vi "main_DMM.vi"() -> ()   [LabVIEW 2018]
uses:
  <instrlib>/Keithley 622x LV 2009/Configure/Source/Typedefs/KE622x -- Voltage Limit.ctl
  <instrlib>/Keithley 622x LV 2009/Configure/Output/Typedefs/KE6221 -- Output Response.ctl
  <instrlib>/Keithley 622x LV 2009/Utility/Typedefs/KE622x -- Instrument Type.ctl
  <instrlib>/Keithley 622x LV 2009/Typedefs/KE622x -- On Off Control.ctl
  <instrlib>/Keithley 622x LV 2009/Configure/Source/Typedefs/KE622x -- Current Range.ctl
  <instrlib>/Keithley 622x LV 2009/Configure/Source/Typedefs/KE622x -- Current Ranges.ctl
  <instrlib>/Keithley 622x LV 2009/Configure/Source/Typedefs/KE622x -- Current Level.ctl
  <vilib>/Utility/file.llb/Write Delimited Spreadsheet (string).vi
  <instrlib>/Keithley 622x LV 2009/Keithley 622x.lvlib
  <instrlib>/Keithley 3706/Keithley 3700 Series.lvlib
panel:
  in  "Measure Count (10)":u32=10 min=1
  in  "Function (2: DC Volts)":T1(ring)=enum."DC Volts"
  out "Measurements":dbl[](array[numeric]) format="%#_6e"
  in  "Timeout (30000 milliseconds)":u32=30000
  in  "file path (dialog if empty)":path
  in  "UnGuarded/ Guarded":enum32{"UnGuarded", "Guarded"}(radio)
  in  "VanderPaw/ Hall Effect":enum32{"Van der Paw", "Hall Effect"}(radio)
  in  "VISA Switch":refnum<visa-resource-name>="GPIB::6"
  out "Close Channel List":string
  out "Iteration number":i32
  out "Current  (A)":dbl
  out "Mean Voltage  (V1-V8)":dbl
  in  "Step Size":T2=0.001 min=-0.105 max=0.105 format="%.4p"
  in  "End":T2=0.001 min=-0.105 max=0.105 format="%.4p"
  in  "Start":T2=0.001 min=-0.105 max=0.105 format="%.4p"
  in  "Turn Off Output If Voltage Limit?":bool=TRUE
  out "Interlock Tripped?":bool
  out "Voltage Limit?":bool
  in  "Check For SCPI Errors? (T)":bool=TRUE
  in  "Current Range In":T3={"Auto Range?"=TRUE, "Man / Selected\nRange"=enum."2nA"}
  in  "Analog Filter State":T5
  in  "Output Response":T6=enum."Slow"
  in  "Voltage Limit (V)":T7=10.0 min=0.1 max=105.0 step=0.01 format="%.2p"
  out "error at Current off":errorcluster
  out "error at current On":errorcluster
  in  "VISA resource dc ac current source (16)":refnum<visa-resource-name>
  out "Configuration Error":errorcluster
  in  "array":dbl[](array[numeric])
  out "output array":dbl[](array[numeric])
  in  "Instrument Type 2":T8=enum."KE6221"
  # "( select : GPIB0::16::INSTR )"
  # "( select : USB0::0x05E6::0x2450::04345639::INSTR )"
  # "( select : USB0::0x05E6::0x3706::04368238::INSTR )"
  # "SYSTEM SWITCH DMM"
types:
  T1 = enum16{"None", "DC Volts", "AC Volts", "DC Current", "AC Current", "2-Wire Ohms", "4-Wire Ohms", "Temperature", "Period", "Frequency", "Continuity", "Commonside Ohms"}
  T2 = typedef "Keithley 622x.lvlib/KE622x -- Current Level.ctl" = dbl
  T3 = typedef "Keithley 622x.lvlib/KE622x -- Current Range.ctl" = cluster{"Auto Range?":bool, "Man / Selected\nRange":T4}
  T4 = typedef "Keithley 622x.lvlib/KE622x -- Current Ranges.ctl" = enum16{"2nA", "20nA", "200nA", "2uA", "20uA", "200uA", "2mA", "20mA", "100mA"}
  T5 = typedef "Keithley 622x.lvlib/KE622x -- On Off Control.ctl" = enum16{"Off", "On"}
  T6 = typedef "Keithley 622x.lvlib/KE6221 -- Output Response.ctl" = enum16{"Fast", "Slow"}
  T7 = typedef "Keithley 622x.lvlib/KE622x -- Voltage Limit.ctl" = dbl
  T8 = typedef "Keithley 622x.lvlib/KE622x -- Instrument Type.ctl" = enum16{"KE6220", "KE6221"}
  T9 = enum16{"Close", "Close Exclusive", "Close Slot Exclusive", "Open", "Open All"}
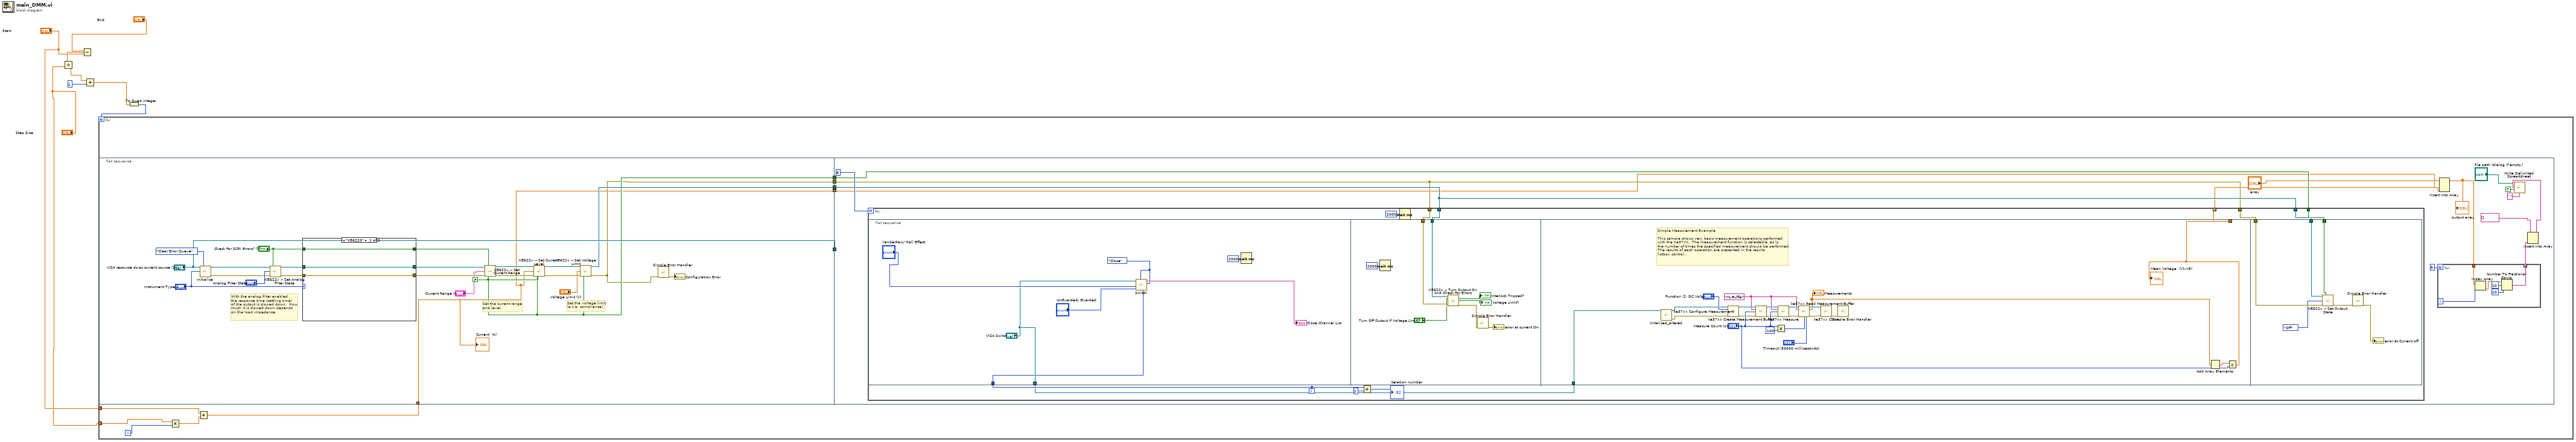
[diagram p0: block diagram]
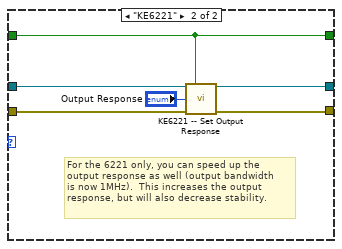
[diagram p2: hidden frame]
diagram:
  n1 = Subtract(x="End", y="Start") -> (x-y=w8:T2)
  n2 = Divide(x=w8, y="Step Size") -> (x/y=w4:T2)
  n3 = Add(x=w4, y=1) -> (x+y=w2:T2)
  n4 = To Quad Integer(1:w2) -> (0:w1:i64)
  n5 = for {
    N: w1 -> [_]
    tunnel: "Step Size" -> [w13]
    tunnel: "Start" -> [w12]
    i -> [w9]
    n6 = flat-sequence {
      tunnel: ["VISA resource dc ac current source (16)"] -> w18
      tunnel: [w22] -> w17
      tunnel: [w20] -> w16
      tunnel: [w21] -> w15
      tunnel: [w19] -> w14
      tunnel: w11 -> [w19]
      tunnel: w18 -> [_]
      tunnel: w17 -> [w63]
      tunnel: w16 -> [w62]
      tunnel: w15 -> [w61]
      tunnel: w14 -> [w52]
      frame #0 {
        w29 = FALSE ("Read Back Set Values? (T)")
        # "Set the voltage limit\n(a.k.a. compliance)."
        # "Set the current range\nand level."
        # "With the analog filter enabled,\nthe response time (settling time)\nof the output is slowed down.  How\nmuch it is slowed down depends\non the load impedance."
        n7 = call <instrlib>:"Initialize.vi"("VISA resource name"="VISA resource dc ac current source (16)", "Error Queue Option"=enum16{"Clear Error Queue", "Error Query"}."Clear Error Queue", "Instrument Type"="Instrument Type 2") -> ("VISA resource name out"=w39:refnum<visa-resource-name>, "error out"=w38:errorcluster)  [unwired: 11 in]
        n8 = call <instrlib>:"KE622x -- Set Analog Filter State.vi"("Resource In"=w39, "Check For SCPI Errors? (T)"="Check For SCPI Errors? (T)", "Analog Filter State"="Analog Filter State", "error in (no error)"=w38) -> ("Resource Out (dupl)"=w37:refnum<visa-resource-name>, "error out"=w35:errorcluster)  [unwired: 10 in]
        n9 = case shown="\"KE6220\"" "Instrument Type 2" {
          tunnel: w37 -> [w43 w50]
          tunnel: w35 -> [w42 w48]
          tunnel: [w43 w47] -> w32
          tunnel: "Check For SCPI Errors? (T)" -> [w44 w46]
          tunnel: [w44 w46] -> w21
          tunnel: [w42 w45] -> w33
          frame "KE6220" {
          }
          frame "KE6221" {
            # "For the 6221 only, you can speed up the\noutput response as well (output bandwidth\nis now 1MHz).  This increases the output\nresponse, but will also decrease stability."
            n10 = call <instrlib>:"KE6221 -- Set Output Response.vi"("Resource In"=w50, "Check For SCPI Errors? (T)"=w46, "KE6221 Output Response"="Output Response", "error in (no error)"=w48) -> ("Resource Out (dupl)"=w47:refnum<visa-resource-name>, "error out"=w45:errorcluster)  [unwired: 10 in]
          }
        }
        n11 = call <instrlib>:"KE622x -- Set Current Range.vi"("Resource In"=w32, "Check For SCPI Errors? (T)"=w21, "Current Range In"="Current Range In", "error in (no error)"=w33, "Read Back Set Values? (T)"=w29) -> ("Resource Out (dupl)"=w31:refnum<visa-resource-name>, "error out"=w30:errorcluster)  [unwired: 8 in, 1 out]
        n12 = call <instrlib>:"KE622x -- Set Current Level.vi"("Resource In"=w31, "Check For SCPI Errors? (T)"=w21, "Current Level (A) In"=w19, "error in (no error)"=w30, "Read Back Set Value? (T)"=w29) -> ("Resource Out (dupl)"=w28:refnum<visa-resource-name>, "error out"=w27:errorcluster)  [unwired: 8 in, 1 out]
        n13 = call <instrlib>:"KE622x -- Set Voltage Limit.vi"("Resource In"=w28, "Check For SCPI Errors? (T)"=w21, "Voltage Limit (V)"="Voltage Limit (V)", "error in (no error)"=w27) -> ("Resource Out (dupl)"=w22:refnum<visa-resource-name>, "error out"=w20:errorcluster)  [unwired: 10 in]
        n14 = call <vilib>:"Simple Error Handler.vi"("error in (no error)"=w20) -> ("error out"=→"Configuration Error":errorcluster)  [unwired: 4 in, 4 out]
        "Current  (A)" <- w19
      }
      frame #1 {
        n15 = for {
          N: 8 -> [_]
          tunnel: [w81] -> w53 mode=indexing
          tunnel: w63 -> [w80]
          tunnel: w62 -> [w79]
          tunnel: w63 -> [w78]
          tunnel: w62 -> [w77]
          tunnel: w61 -> [w76]
          i -> [w74]
          n16 = flat-sequence {
            tunnel: w74 -> [w89]
            tunnel: ["VISA Switch"] -> w72
            tunnel: w80 -> [w97]
            tunnel: w79 -> [w96]
            tunnel: [w117] -> w81
            tunnel: w72 -> [w99]
            tunnel: w78 -> [w124]
            tunnel: w77 -> [w123]
            tunnel: w76 -> [w119]
            frame #0 {
              w86 = T9."Close" ("Operation 3")
              n17 = call "Switch.vi"("Numeric"=w89, "Operation 2"=w86, "UnGuarded/ Guarded"="UnGuarded/ Guarded", "Radio Buttons"="VanderPaw/ Hall Effect", "Operation 3"=w86, "VISA Refnum in"="VISA Switch") -> ("Close Channel List 2"=→"Close Channel List":string)  [unwired: 5 in]
              n18 = Wait (ms)(milliseconds to wait=u32 2000) -> ()  [unwired: 1 out]
            }
            frame #1 {
              n19 = Wait (ms)(milliseconds to wait=u32 2000) -> ()  [unwired: 1 out]
              n20 = call <instrlib>:"KE622x -- Turn Output On And Check For Errors.vi"("Resource In"=w97, "Turn Off Output If Compliance?"="Turn Off Output If Voltage Limit?", "error in (no error)"=w96) -> ("Interlock Tripped?"=→"Interlock Tripped?":bool, "Compliance?"=→"Voltage Limit?":bool, "error out"=w91:errorcluster)  [unwired: 9 in, 1 out]
              n21 = call <vilib>:"Simple Error Handler.vi"("error in (no error)"=w91) -> ("error out"=→"error at current On":errorcluster)  [unwired: 4 in, 4 out]
            }
            frame #2 {
              w108 = "MyBuffer" ("Buffer Name")
              # "Simple Measurement Example\n \nThis sample shows very basic measurement operations performed\nwith the Ke37XX.  The measurement function is selectable, as is\nthe number of times the specified measurement should be performed.\nThe results of each operation are presented in the results\nlistbox control."
              n22 = call "Initalized_altered.vi"("VISA Refnum in"=w99) -> ("error out"=w100:errorcluster, "VISA Refnum out"=w101:refnum<visa-resource-name>)  [unwired: 9 in]
              n23 = call <instrlib>:"ke37xx Configure Measurement.vi"("VISA Resource Name"=w101, "Function (0: None)"="Function (2: DC Volts)", "error in (no error)"=w100) -> ("VISA Resource Name Out"=w113:refnum<visa-resource-name>, "error out"=w112:errorcluster)  [unwired: 11 in]
              n24 = call <instrlib>:"ke37xx Create Measurement Buffer.vi"("VISA Resource Name"=w113, "Buffer Name"=w108, "Capacity"="Measure Count (10)", "error in (no error)"=w112) -> ("VISA Resource Name Out"=w111:refnum<visa-resource-name>, "error out"=w98:errorcluster)  [unwired: 10 in]
              n25 = Multiply(x="Measure Count (10)", y=u32 100) -> (x*y=w105:u32)
              n26 = call <instrlib>:"ke37xx Measure.vi"("VISA Resource Name"=w111, "Buffer Name"=w108, "Measure Count (1)"="Measure Count (10)", "error in (no error)"=w98) -> ("VISA Resource Name Out"=w110:refnum<visa-resource-name>, "error out"=w109:errorcluster)  [unwired: 7 in, 3 out]
              n27 = call <instrlib>:"ke37xx Read Measurement Buffer.vi"("VISA Resource Name"=w110, "Buffer Name"=w108, "error in (no error)"=w109, "Bytes To Read (1024)"=w105, "Timeout (10 seconds)"="Timeout (30000 milliseconds)") -> ("VISA Resource Name Out"=w116:refnum<visa-resource-name>, "Readings"=w103:dbl[], "error out"=w106:errorcluster)  [unwired: 4 in, 4 out]
              "Measurements" <- w103
              n28 = call <instrlib>:"ke37xx Close.vi"("VISA resource name"=w116, "error in (no error)"=w106) -> ("error out"=w115:errorcluster)  [unwired: 13 in]
              n29 = call <vilib>:"Simple Error Handler.vi"("error in (no error)"=w115) -> ()  [unwired: 1 in, 8 out]
              n30 = Add Array Elements(numeric array=w103) -> (sum=w118:dbl)
              n31 = Divide(x=w118, y="Measure Count (10)") -> (x/y=w117:dbl)
              "Mean Voltage  (V1-V8)" <- w117
            }
            frame #3 {
              n32 = call <instrlib>:"KE622x -- Set Output State.vi"("Resource In"=w124, "Check For SCPI Errors? (T)"=w119, "Output State"=KE622x_--_On_Off_Control."Off", "error in (no error)"=w123) -> ("error out"=w120:errorcluster)  [unwired: 10 in, 1 out]
              n33 = call <vilib>:"Simple Error Handler.vi"("error in (no error)"=w120) -> ("error out"=→"error at Current off":errorcluster)  [unwired: 4 in, 4 out]
            }
          }
          n34 = Add(x=w74, y=1) -> (x+y=→"Iteration number":i32)
          n35 = Wait (ms)(milliseconds to wait=u32 2000) -> ()  [unwired: 1 out]
        }
        n36 = Insert Into Array(array="array", new element #1=w52, new element #2=w53) -> (w58:dbl[])  [unwired: 1 in]
        "output array" <- w58
        n37 = for {
          N: 9 -> [_]
          tunnel: w58 -> [w71]
          tunnel: [w68] -> w57 mode=indexing
          i -> [w70]
          n38 = Index Array(array=w71, index=w70) -> (element=w69:dbl)
          n39 = Number To Fractional String(number=w69, width (-)=i16 10, precision (6)=i16 10) -> (F-format string=w68:string)  [unwired: 1 in]
        }
        n40 = Insert Into Array(array=string[] [], new element=w57) -> (w55:string[])  [unwired: 1 in]
        n41 = call-poly <vilib>:"Write Delimited Spreadsheet.vi"("file path (dialog if empty)"="file path (dialog if empty)", "1D data"=w55, "append to file? (new file:F)"=TRUE, "delimiter (\\t)"="," ("delimiter (\\t)")) -> ()  [unwired: 10 in, 2 out]
      }
    }
    n42 = Multiply(x=w13, y=w9) -> (x*y=w10:T2)
    n43 = Add(x=w12, y=w10) -> (x+y=w11:T2)
  }
